vi "Register Generic Sink as Default.vi"(8 "error in (no error)":errorcluster, 11 "Sink":refnum<class "Sink.lvclass">) -> (0 "error out":errorcluster)   [LabVIEW 2020, in "LV Log.lvlib"]
uses:
  LV Log.lvlib
  Sink/Sink.lvclass
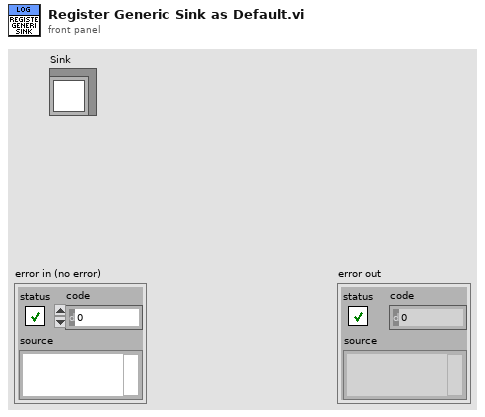
[diagram p1: front panel]
types:
  T1 = enum16{"Init", "Get Logger", "Register Sink", "Set Global Debug Level", "Get Sinks"}
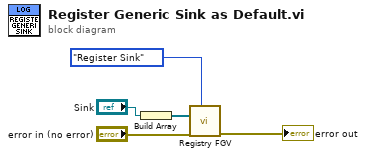
[diagram p0: block diagram]
diagram:
  n1 = Build Array("Sink") -> (w2:refnum<class "Sink.lvclass">[])
  n2 = call "Registry FGV.vi"("State (Get Logger)"=T1."Register Sink", "error in (no error)"="error in (no error)", "Sink(s)"=w2) -> ("error out"=→"error out":errorcluster)  [unwired: 5 in, 3 out]
